vi "Compute DistanceToBalls.vi"(6 "Target Width (in)":dbl=6.5 format="%.1f", 8 "results":T1, 10 "FOV":dbl=68.5, 11 "Image Src":T2) -> (0 "results out":T1, 1 "Off Angle":dbl, 3 "Image Dst Out":T2, 4 "Distance":dbl)   [LabVIEW 2023]
doc: "Using the camera lens information and the real world size of the target, use trig and ratios to determine the distance to the target. Also returns the location relative to the image center in a (-1 , 1) coordinate system that may be useful for steering the robot."
uses:
  <vilib>/vision/Image Controls.llb/IMAQ Image.ctl
  Target Fields.ctl
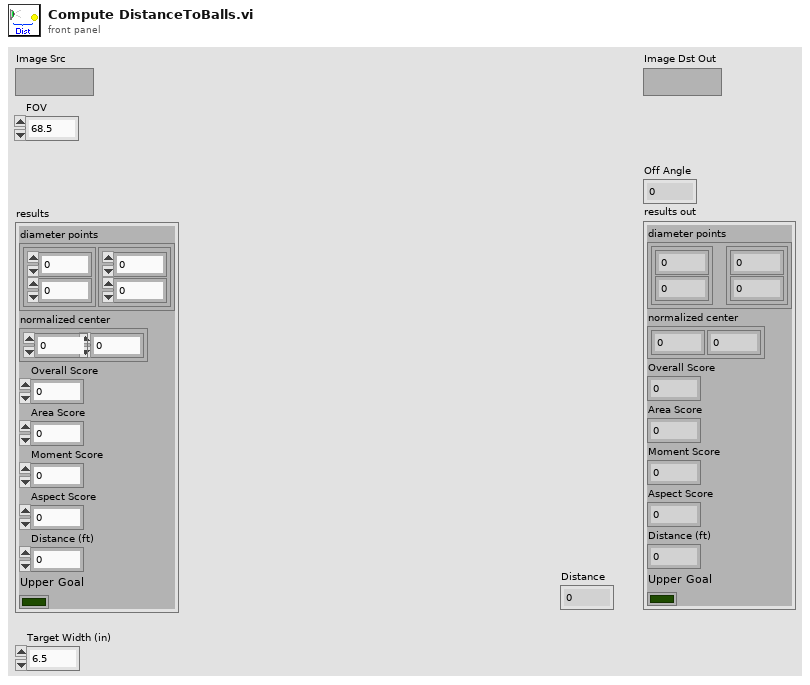
[diagram p1: front panel]
types:
  T1 = typedef "Target Fields.ctl" = cluster{"diameter points":cluster{"first point":cluster{"x":dbl, "y":dbl}, "projected point":cluster{"x":dbl, "y":dbl}}, "normalized center":cluster{"x":dbl, "y":dbl}, "Overall Score":dbl, "Area Score":dbl, "Moment Score":dbl, "Aspect Score":dbl, "Distance (ft)":dbl, "Upper Goal":bool}
  T2 = typedef "IMAQ Image.ctl" = refnum<image>
  T3 = cluster{"first point":cluster{"x":dbl, "y":dbl}, "projected point":cluster{"x":dbl, "y":dbl}}
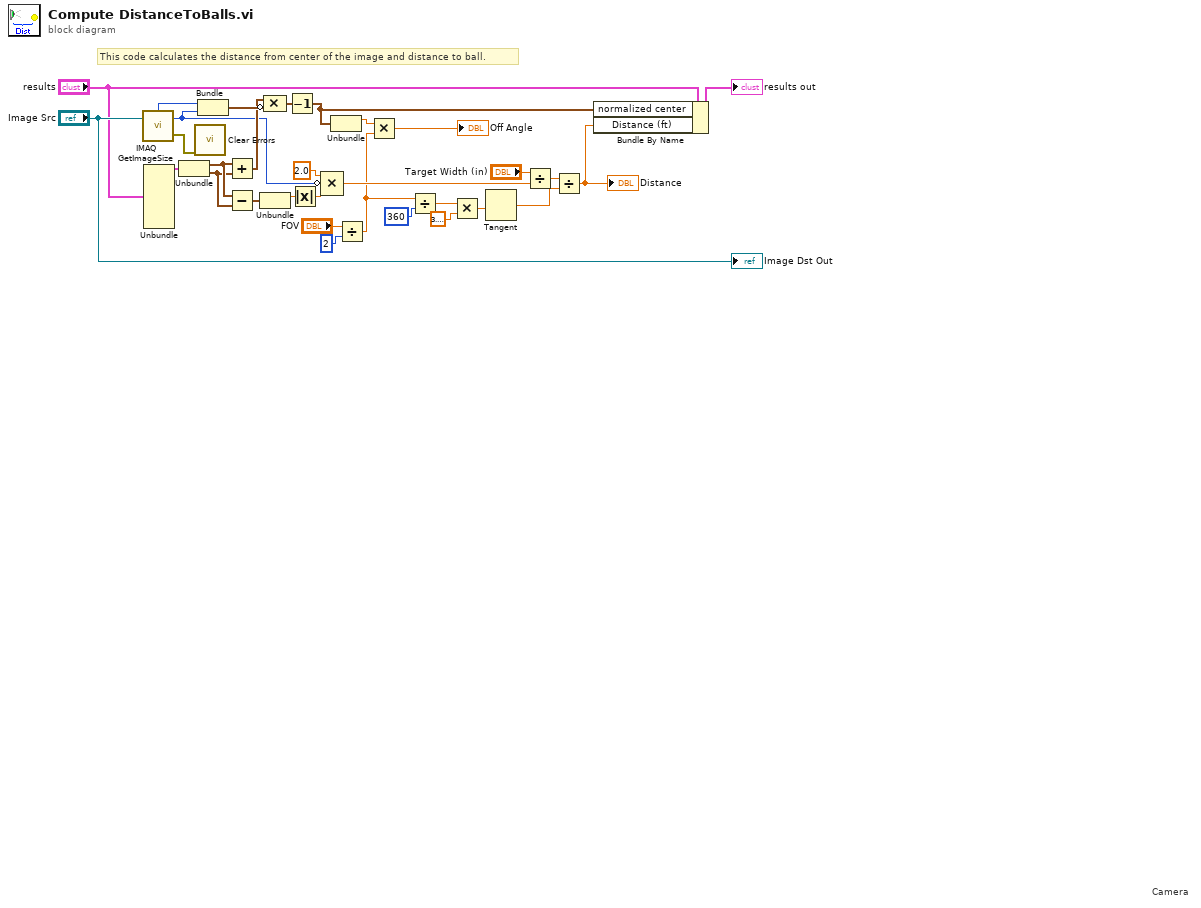
[diagram p0: block diagram]
diagram:
  # "Camera"
  # "This code calculates the distance from center of the image and distance to ball."
  n1 = call "IMAQ GetImageSize"("Image"="Image Src") -> ("Y Resolution"=w12:i32, "X Resolution"=w9:i32, "error out"=w23:errorcluster)  [unwired: 3 in]
  n2 = Unbundle("results") -> ("diameter points"=w1:T3)  [unwired: 7 out]
  n3 = Unbundle(w1) -> ("first point"=w15:cluster{"x":dbl, "y":dbl}, "projected point"=w14:cluster{"x":dbl, "y":dbl})
  n4 = call <vilib>:"Clear Errors.vi"("error in (no error)"=w23) -> ()  [unwired: 5 in, 2 out]
  n5 = Bundle("X Resolution"=w9, "Y Resolution"=w12) -> (w16:cluster{"X Resolution":i32, "Y Resolution":i32})  [unwired: 1 in]
  n6 = Add(x=w15, y=w14) -> (x+y=w13:cluster{"x":dbl, "y":dbl})
  n7 = Subtract(x=w15, y=w14) -> (x-y=w20:cluster{"x":dbl, "y":dbl})
  n8 = Unbundle(w20) -> ("x"=w19:dbl)  [unwired: 1 out]
  n9 = Compound Arithmetic op=MULTIPLY(w13, invert w16) -> (w4:cluster{dbl, dbl})
  n10 = Decrement(x=w4) -> (x-1=w10:cluster{dbl, dbl})
  n11 = Absolute Value(x=w19) -> (abs(x)=w21:dbl)
  n12 = Compound Arithmetic op=MULTIPLY(2.0, invert w12, w21) -> (w24:dbl)
  n13 = Unbundle(w10) -> (w8:dbl)  [unwired: 1 out]
  n14 = Divide(x="FOV", y=2) -> (x/y=w3:dbl)
  n15 = Multiply(x=w8, y=w3) -> (x*y=→"Off Angle":dbl)
  n16 = Divide(x=w3, y=360) -> (x/y=w28:dbl)
  n17 = Multiply(x=w28, y=3.141592653589793) -> (x*y=w29:dbl)
  n18 = Tangent(1:w29) -> (0:w26:dbl)
  n19 = Divide(x="Target Width (in)", y=w24) -> (x/y=w7:dbl)
  n20 = Divide(x=w7, y=w26) -> (x/y=w6:dbl)
  "Distance" <- w6
  n21 = Bundle By Name(cluster="results", "normalized center"=w10, "Distance (ft)"=w6) -> (→"results out":T1)
  "Image Dst Out" <- "Image Src"
